vi "Velocity mMc Edited.vi"(0 "velocity in":dbl, 1 "Port":T1={"P type"=0, "reference"="", " Terminator "="\r\n", "Timeout"=300} {"Timeout" step=10; "P type" items=["none", "RS-232C"]}, 3 "error in (no error)":errorcluster, 4 "set/get":bool caption="set\n\n\nget", 5 "Controller #":string) -> (6 "velocity out":dbl, 9 "error out":errorcluster)   [LabVIEW 2021]
panel:
  # "Velocity"
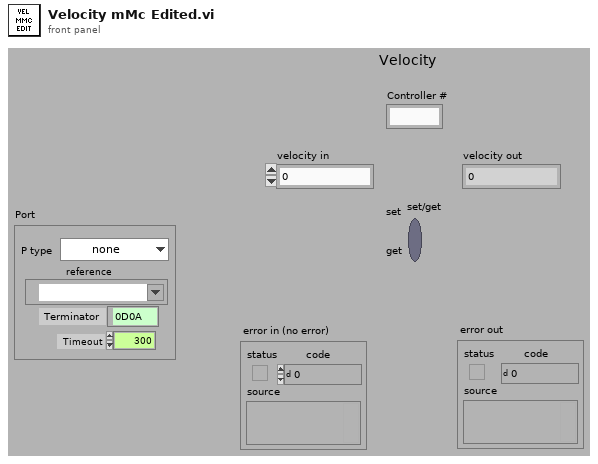
[diagram p1: front panel]
types:
  T1 = cluster{"P type":u16, "reference":refnum<visa-resource-name>, " Terminator ":string, "Timeout":i32}
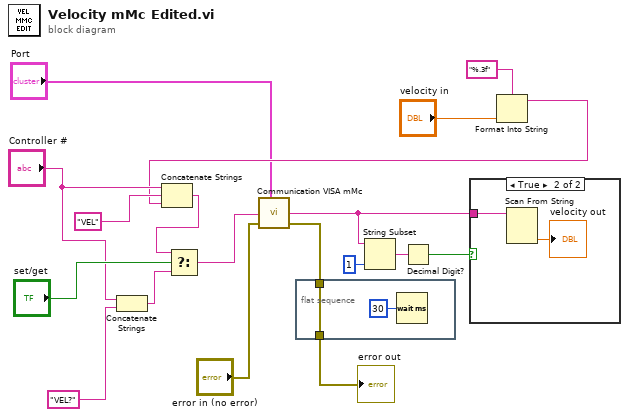
[diagram p0: block diagram]
diagram:
  n1 = Concatenate Strings("Controller #", "VEL?") -> (w18:string)
  n2 = flat-sequence {
    tunnel: w2 -> [w20]
    tunnel: [w20] -> w1
    frame #0 {
      n3 = Wait (ms)(milliseconds to wait=u32 30) -> ()  [unwired: 1 out]
    }
  }
  n4 = Format Into String(format string="%.3f", "velocity in") -> (resulting string=w8:string)  [unwired: 2 in, 1 out]
  n5 = Concatenate Strings("Controller #", "VEL", w8) -> (w16:string)
  n6 = Select(t=w16, s="set/get", f=w18) -> (s? t:f=w15:string)
  n7 = call "Communication VISA mMc.vi"("Port"="Port", "Command"=w15, "error in (no error)"="error in (no error)") -> ("Return"=w4:string, "error out"=w2:errorcluster)  [unwired: 3 in, 2 out]
  n8 = String Subset(string=w4, length (rest)=1 ("length (rest)")) -> (substring=w6:string)  [unwired: 1 in]
  n9 = Decimal Digit?(1:w6) -> (0:w5:bool)
  n10 = case shown="True" w5 {
    tunnel: w4 -> [_ w21]
    frame False {
    }
    frame True {
      n11 = Scan From String(input string=w21) -> (output 1=→"velocity out":dbl)  [unwired: 4 in, 3 out]
    }
  }
  "error out" <- w1
